vi "ElapsedTime_FGV.vi"(7 "Command":T1, 8 "Error In":errorcluster, 11 "DesiredTime (s)":u32) -> (0 "Error Out":errorcluster, 2 "Done?":bool, 3 "ElapsedTime":dbl)   [LabVIEW 2017]
doc: "This is a Functional Global Variable that keeps track of the elapsed time since the last START command was sent."
uses:
  Controls/ElapsedTimeCommand.ctl
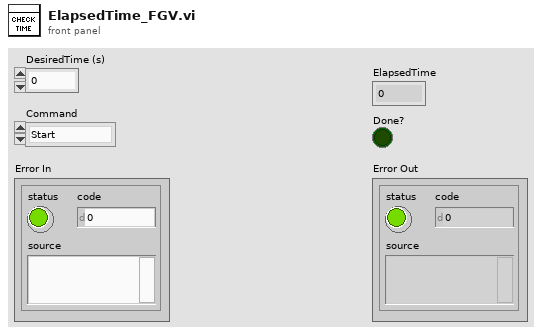
[diagram p1: front panel]
types:
  T1 = typedef "ElapsedTimeCommand.ctl" = enum16{"Start", "CheckTime", "Stop"}
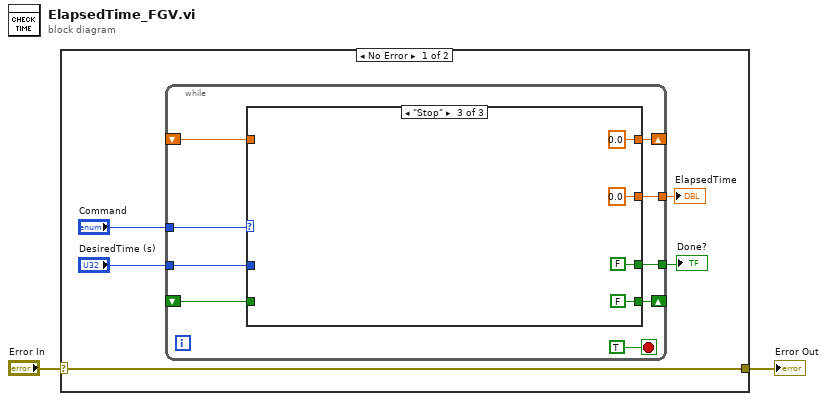
[diagram p0: block diagram]
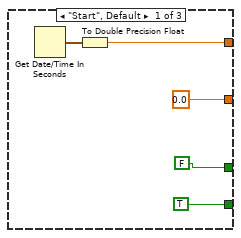
[diagram p2: hidden frame]
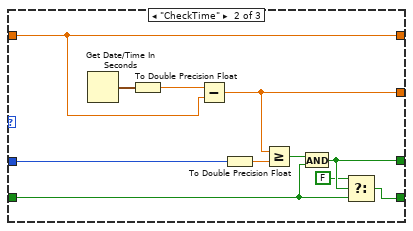
[diagram p3: hidden frame]
diagram:
  n1 = case shown="No Error" "Error In" {
    selector: "Error In" -> [w4 w37]
    tunnel: [w4 w37] -> w1
    frame No Error {
      n2 = while {
        shift-right: [w14] -> _
        shift-left: _ -> [w13]
        tunnel: "Command" -> [w15]
        tunnel: [w12] -> w7
        tunnel: "DesiredTime (s)" -> [w11]
        tunnel: [w10] -> w5
        shift-right: [w9] -> _
        shift-left: _ -> [w8]
        stop <- TRUE stop-if-true
        n3 = case shown="\"Stop\"" w15 {
          tunnel: [w20 w30 0.0] -> w14
          tunnel: w13 -> [_ w30 _]
          tunnel: [0.0 w29 0.0] -> w12
          tunnel: w11 -> [_ w27 _]
          tunnel: [FALSE w25 FALSE] -> w10
          tunnel: [TRUE w22 FALSE ("t")] -> w9
          tunnel: w8 -> [_ w24 _]
          frame "Start", Default {
            n4 = Get Date/Time In Seconds() -> (seconds since 1Jan1904=w21:timestamp)
            n5 = To Double Precision Float(number=w21) -> (double precision float=w20:dbl)
          }
          frame "CheckTime" {
            n6 = Get Date/Time In Seconds() -> (seconds since 1Jan1904=w32:timestamp)
            n7 = To Double Precision Float(number=w32) -> (double precision float=w31:dbl)
            n8 = Subtract(x=w31, y=w30) -> (x-y=w29:dbl)
            n9 = To Double Precision Float(number=w27) -> (double precision float=w28:dbl)
            n10 = Greater Or Equal?(x=w29, y=w28) -> (x >= y?=w26:bool)
            n11 = And(x=w26, y=w24) -> (x .and. y?=w25:bool)
            n12 = Select(t=FALSE, s=w25, f=w24) -> (s? t:f=w22:bool)
          }
          frame "Stop" {
          }
        }
      }
      "ElapsedTime" <- w7
      "Done?" <- w5
    }
    frame Error {
    }
  }
  "Error Out" <- w1
